vi "CR-Initial CameraCCD6.vi"(8 "error in (no error)":errorcluster caption="错误输入（无错误）") -> (0 "error out":errorcluster caption="错误输出", 3 "Session Out":T1)   [LabVIEW 2017]
uses:
  <vilib>/userdefined/High Color/IMAQdx.ctl
  <vilib>/vision/driver/IMAQdx.llb/IMAQdx Acquisition Mode.ctl
  <vilib>/vision/driver/NI_Vision_Acquisition_Software.lvlib
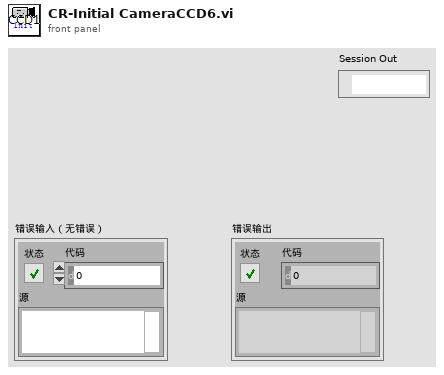
[diagram p1: front panel]
types:
  T1 = typedef "IMAQdx.ctl" = refnum<k21>
  T2 = typedef "NI_Vision_Acquisition_Software.lvlib/IMAQdx Acquisition Mode.ctl" = enum32{"One Shot", "Continuous"}
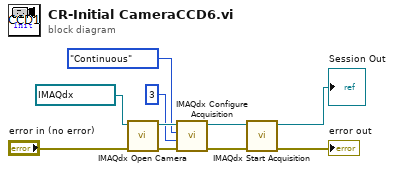
[diagram p0: block diagram]
diagram:
  n1 = call <vilib>:"IMAQdx Open Camera.vi"("error in"="error in (no error)", "Session In"=T1 "cam0") -> ("error out"=w7:errorcluster, "Session Out"=w10:T1)  [unwired: 8 in]
  n2 = call <vilib>:"IMAQdx Configure Acquisition.vi"("error in"=w7, "Number of Buffers"=u32 3, "Continuous?"=IMAQdx_Acquisition_Mode."Continuous", "Session In"=w10) -> ("error out"=w3:errorcluster, "Session Out"=w4:T1)  [unwired: 6 in]
  n3 = call <vilib>:"IMAQdx Start Acquisition.vi"("error in"=w3, "Session In"=w4) -> ("error out"=→"error out":errorcluster, "Session Out"=→"Session Out":T1)  [unwired: 8 out]
